vi "load_txt.vi"(8 "error in (no error)":errorcluster, 11 "Path":path) -> (0 "error out":errorcluster, 3 "Data":dbl[](array[numeric]))   [LabVIEW 2024]
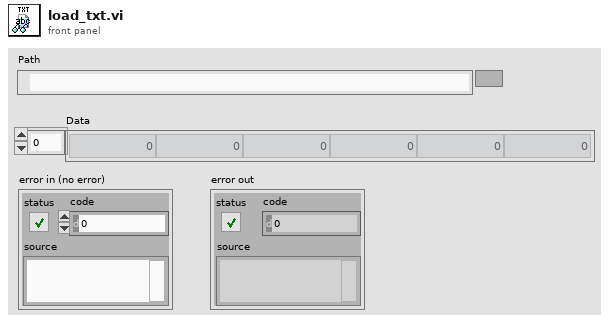
[diagram p1: front panel]
types:
  T1 = enum16{"open", "replace", "create", "open or create", "replace or create", "replace or create with confirmation"}
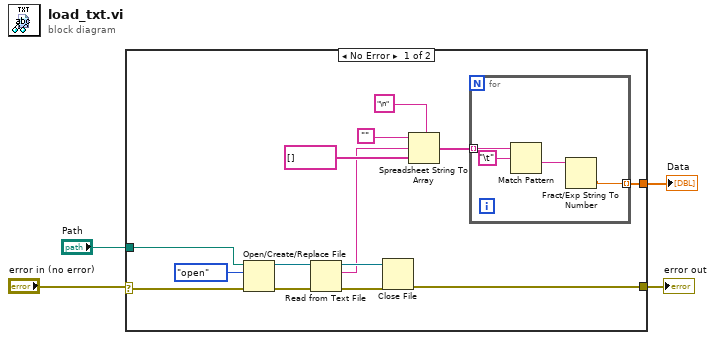
[diagram p0: block diagram]
diagram:
  n1 = case shown="No Error" "error in (no error)" {
    selector: "error in (no error)" -> [w18 w23]
    tunnel: "Path" -> [w15 _]
    tunnel: [w11 _] -> w2
    tunnel: [w10 w23] -> w1
    frame No Error {
      n2 = Open/Create/Replace File(file path (use dialog)=w15, error in=w18, operation (0:open)=T1."open") -> (refnum out=w14:refnum<file>, error out=w17:errorcluster)  [unwired: 3 in, 1 out]
      n3 = Read from Text File(file (use dialog)=w14, error in=w17) -> (refnum out=w13:refnum<file>, text=w6:string, error out=w16:errorcluster)  [unwired: 2 in, 1 out]
      n4 = Close File(refnum=w13, error in=w16) -> (error out=w10:errorcluster)  [unwired: 1 out]
      n5 = Spreadsheet String To Array(delimiter (Tab)="\n", format string="", spreadsheet string=w6, array type (2D Dbl)=string[] []) -> (array=w8:string[])
      n6 = for {
        tunnel: [w20] -> w11 mode=indexing
        tunnel: w8 -> [w19] mode=indexing
        n7 = Match Pattern(string=w19, regular expression="\t") -> (after substring=w21:string)  [unwired: 1 in, 3 out]
        n8 = Fract/Exp String To Number(string=w21) -> (number=w20:dbl)  [unwired: 3 in, 1 out]
      }
    }
    frame Error {
    }
  }
  "error out" <- w1
  "Data" <- w2
